vi "VD-Disconnect.vi"(8 "error in (no error)":errorcluster, 11 "VD-LV-LiteVNA in":refnum<class "VD-LV-LiteVNA.lvclass">) -> (0 "error out":errorcluster, 3 "VD-LV-LiteVNA out":refnum<class "VD-LV-LiteVNA.lvclass">)   [LabVIEW 2020, in "VD-LV-LiteVNA.lvclass"]
uses:
  VD-LV-LiteVNA.lvclass
  VD-LV-LiteVNA.lvclass/VD-LV-LiteVNA.ctl
  hardware-protocol/serial/HP-S-Serial.lvclass
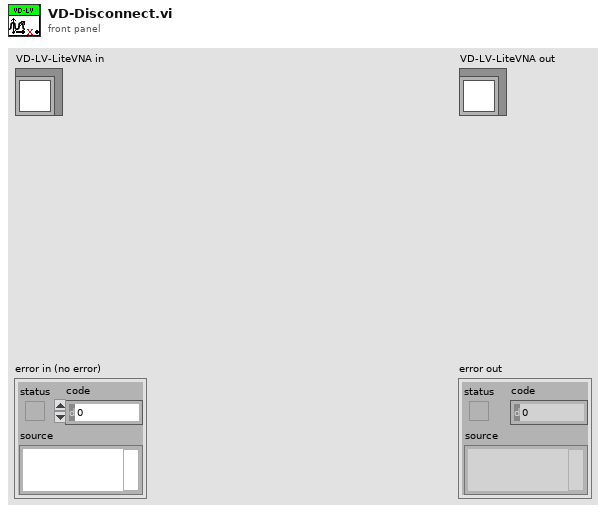
[diagram p1: front panel]
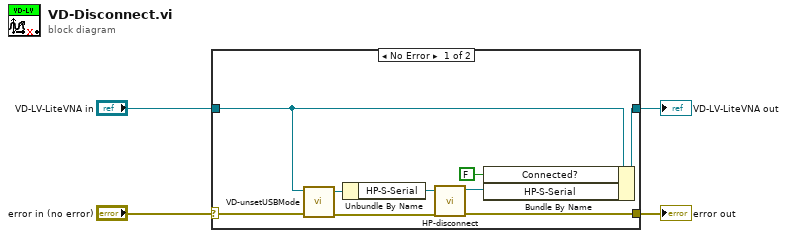
[diagram p0: block diagram]
diagram:
  n1 = case shown="No Error" "error in (no error)" {
    selector: "error in (no error)" -> [w6 w15]
    tunnel: [w13 w15] -> w3
    tunnel: [w12 w14] -> w1
    tunnel: "VD-LV-LiteVNA in" -> [w8 w14]
    frame No Error {
      n2 = call "VD-unsetUSBMode.vi"("error in (no error)"=w6, "VD-LV-LiteVNA in"=w8) -> ("error out"=w5:errorcluster, "VD-LV-LiteVNA out"=w7:refnum<class "VD-LV-LiteVNA.lvclass">)  [unwired: 8 in]
      n3 = Unbundle By Name(w7) -> ("HP-S-Serial"=w10:refnum<class "HP-S-Serial.lvclass">)
      n4 = call-dynamic "HP-disconnect.vi"("error in (no error)"=w5, "HP-S-Serial in"=w10) -> ("error out"=w13:errorcluster, "HP-S-Serial out"=w11:refnum<class "HP-S-Serial.lvclass">)  [unwired: 8 in]
      n5 = Bundle By Name(cluster=w8, "Connected?"=FALSE ("session info.Connected?"), "HP-S-Serial"=w11) -> (w12:refnum<class "VD-LV-LiteVNA.lvclass">)
    }
    frame Error {
    }
  }
  "error out" <- w3
  "VD-LV-LiteVNA out" <- w1
